vi "radio_control.vi"() -> ()   [LabVIEW 2012]
uses:
  <vilib>/Instr/_visa.llb/VISA Configure Serial Port (Instr).vi
panel:
  out "Response":string[](array[string])
  in  "Commands":string[](array[string])
  out "error out":errorcluster
  out "read buffer":string
  in  "VISA resource name":refnum<visa-resource-name>
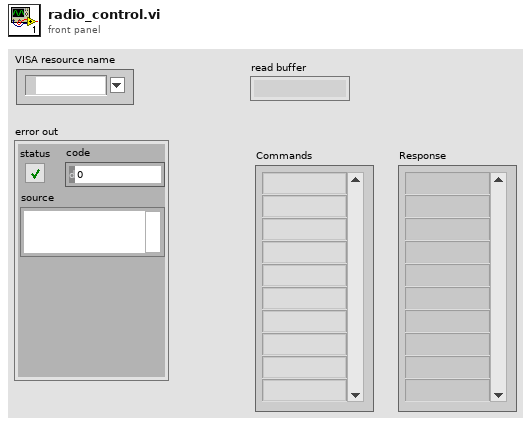
[diagram p1: front panel]
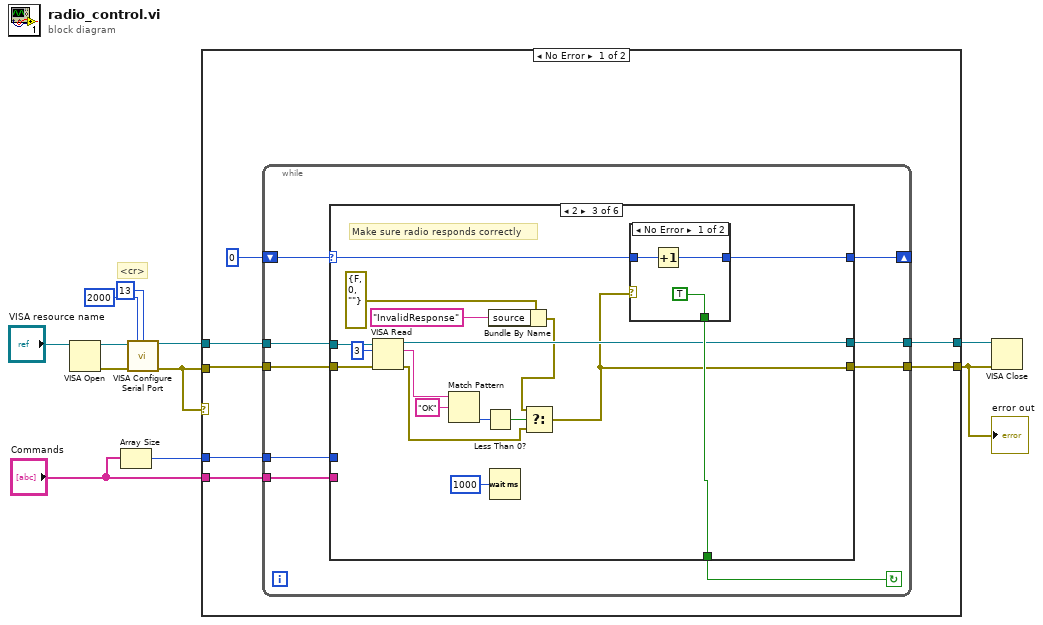
[diagram p0: block diagram]
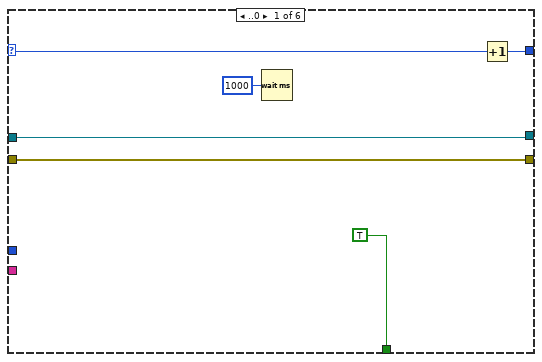
[diagram p2: hidden frame]
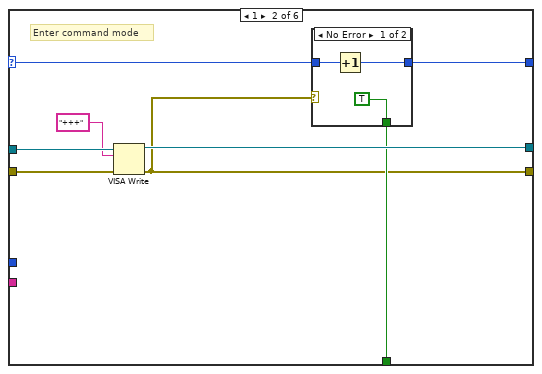
[diagram p3: hidden frame]
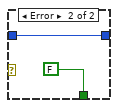
[diagram p4: hidden frame]
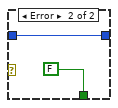
[diagram p5: hidden frame]
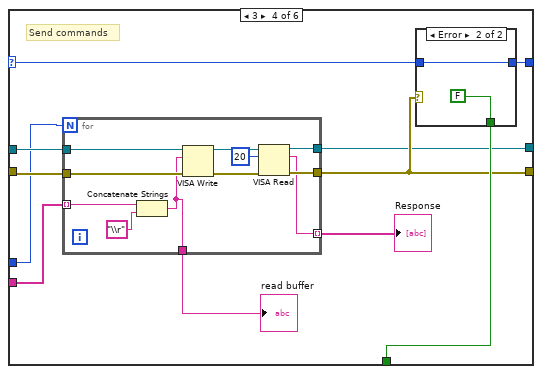
[diagram p6: hidden frame]
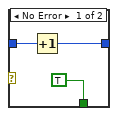
[diagram p7: hidden frame]
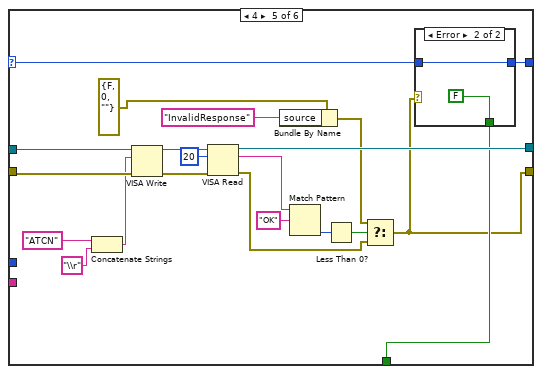
[diagram p8: hidden frame]
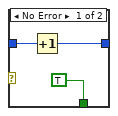
[diagram p9: hidden frame]
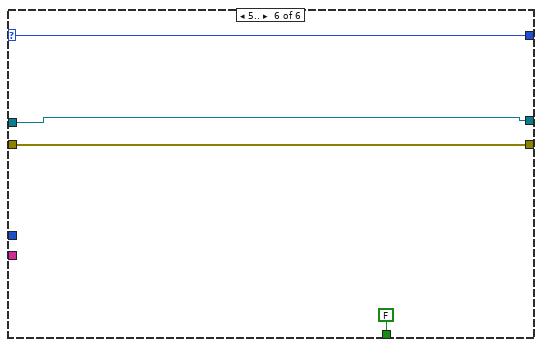
[diagram p10: hidden frame]
diagram:
  # "<cr>"
  n1 = VISA Open(VISA resource name="VISA resource name") -> (VISA resource name=w10:refnum<visa-resource-name>, error out=w9:errorcluster)  [unwired: 4 in]
  n2 = Array Size(array="Commands") -> (size(s)=w1:i32)
  n3 = call-poly "VISA Configure Serial Port"("VISA resource name"=w10, "timeout (10sec)"=u32 2000, "termination char\n(0xA = '\\n' = LF)"=u8 13 ("termination char\n(0xA = '\\n' = LF)"), "error in (no error)"=w9) -> ("VISA resource name out"=w8:refnum<visa-resource-name>, "error out"=w7:errorcluster)  [unwired: 10 in]
  n4 = case shown="No Error" w7 {
    tunnel: w8 -> [w18 w127]
    tunnel: w7 -> [w17 w126]
    tunnel: [w16 w127] -> w6
    tunnel: [w15 w126] -> w5
    tunnel: "Commands" -> [w13 _]
    tunnel: w1 -> [w12 _]
    frame No Error {
      n5 = while {
        tunnel: w18 -> [w27]
        tunnel: w17 -> [w26]
        tunnel: [w25] -> w16
        tunnel: [w24] -> w15
        shift-right: [w22] -> _
        shift-left: 0 -> [w23]
        tunnel: w13 -> [w20]
        tunnel: w12 -> [w19]
        stop <- w21 continue-if-true
        n6 = case shown="2" w23 {
          tunnel: w27 -> [w29 w41 w63 w76 w113 w125]
          tunnel: w26 -> [w28 w40 w61 w75 w112 w124]
          tunnel: [w29 w38 w57 w70 w111 w125] -> w25
          tunnel: [w28 w34 w52 w71 w96 w124] -> w24
          selector: w23 -> [w30 w37 w59 w78 w108 w123]
          tunnel: [w31 w36 w60 w79 w110 w123] -> w22
          tunnel: [TRUE w35 w58 w77 w109 FALSE] -> w21
          tunnel: w20 -> [_ _ _ w74 _ _]
          tunnel: w19 -> [_ _ _ w73 _ _]
          frame ..0 {
            n7 = Wait (ms)(milliseconds to wait=u32 1000) -> ()  [unwired: 1 out]
            n8 = Increment(x=w30) -> (x+1=w31:i32)
          }
          frame 1 {
            # "Enter command mode"
            n9 = VISA Write(VISA resource name=w41, write buffer="+++", error in (no error)=w40) -> (VISA resource name out=w38:refnum<visa-resource-name>, error out=w34:errorcluster)  [unwired: 1 out]
            n10 = case shown="No Error" w34 {
              tunnel: w37 -> [w44 w45]
              tunnel: [w43 w45] -> w36
              tunnel: [TRUE FALSE] -> w35
              frame No Error {
                n11 = Increment(x=w44) -> (x+1=w43:i32)
              }
              frame Error {
              }
            }
          }
          frame 2 {
            # "Make sure radio responds correctly"
            n12 = VISA Read(VISA resource name=w63, byte count=u32 3, error in (no error)=w61) -> (VISA resource name out=w57:refnum<visa-resource-name>, read buffer=w56:string, error out=w51:errorcluster)  [unwired: 1 out]
            n13 = Match Pattern(string=w56, regular expression="OK") -> (offset past match=w54:i32)  [unwired: 1 in, 3 out]
            n14 = Less Than 0?(x=w54) -> (x < 0?=w53:bool)
            n15 = Bundle By Name(cluster=errorcluster {"status"=FALSE, "code"=0, "source"=""} ("error constant"), "source"="InvalidResponse") -> (w48:errorcluster)
            n16 = Wait (ms)(milliseconds to wait=u32 1000) -> ()  [unwired: 1 out]
            n17 = Select(t=w48, s=w53, f=w51) -> (s? t:f=w52:errorcluster)
            n18 = case shown="No Error" w52 {
              tunnel: w59 -> [w66 w67]
              tunnel: [w65 w67] -> w60
              tunnel: [TRUE FALSE] -> w58
              frame No Error {
                n19 = Increment(x=w66) -> (x+1=w65:i32)
              }
              frame Error {
              }
            }
          }
          frame 3 {
            # "Send commands"
            n20 = for {
              N: w73 -> [_]
              tunnel: w76 -> [w89]
              tunnel: w75 -> [w88]
              tunnel: w74 -> [w87] mode=indexing
              tunnel: [w83] -> w71
              tunnel: [w82] -> w72 mode=indexing
              tunnel: [w81] -> w70
              tunnel: [w80] -> w69
              n21 = Concatenate Strings(w87, "\\r" ("string")) -> (w80:string)
              n22 = VISA Write(VISA resource name=w89, write buffer=w80, error in (no error)=w88) -> (VISA resource name out=w86:refnum<visa-resource-name>, error out=w85:errorcluster)  [unwired: 1 out]
              n23 = VISA Read(VISA resource name=w86, byte count=u32 20, error in (no error)=w85) -> (VISA resource name out=w81:refnum<visa-resource-name>, read buffer=w82:string, error out=w83:errorcluster)  [unwired: 1 out]
            }
            "Response" <- w72
            "read buffer" <- w69
            n24 = case shown="Error" w71 {
              tunnel: w78 -> [w93 w94]
              tunnel: [w92 w94] -> w79
              tunnel: [TRUE FALSE] -> w77
              frame No Error {
                n25 = Increment(x=w93) -> (x+1=w92:i32)
              }
              frame Error {
              }
            }
          }
          frame 4 {
            n26 = Concatenate Strings("ATCN" ("string"), "\\r" ("string")) -> (w106:string)
            n27 = VISA Write(VISA resource name=w113, write buffer=w106, error in (no error)=w112) -> (VISA resource name out=w116:refnum<visa-resource-name>, error out=w115:errorcluster)  [unwired: 1 out]
            n28 = VISA Read(VISA resource name=w116, byte count=u32 20, error in (no error)=w115) -> (VISA resource name out=w111:refnum<visa-resource-name>, read buffer=w100:string, error out=w98:errorcluster)  [unwired: 1 out]
            n29 = Bundle By Name(cluster=errorcluster {"status"=FALSE, "code"=0, "source"=""} ("error constant"), "source"="InvalidResponse") -> (w99:errorcluster)
            n30 = Match Pattern(string=w100, regular expression="OK") -> (offset past match=w102:i32)  [unwired: 1 in, 3 out]
            n31 = Less Than 0?(x=w102) -> (x < 0?=w101:bool)
            n32 = Select(t=w99, s=w101, f=w98) -> (s? t:f=w96:errorcluster)
            n33 = case shown="Error" w96 {
              tunnel: w108 -> [w119 w120]
              tunnel: [w118 w120] -> w110
              tunnel: [TRUE FALSE] -> w109
              frame No Error {
                n34 = Increment(x=w119) -> (x+1=w118:i32)
              }
              frame Error {
              }
            }
          }
          frame 5.. {
          }
        }
      }
    }
    frame Error {
    }
  }
  "error out" <- w5
  n35 = VISA Close(VISA resource name=w6, error in (no error)=w5) -> ()  [unwired: 1 out]
